vi "IMAQ OCR.vi"(0 "Image In":T1, 7 "error in":errorcluster) -> (21 "String (OCR/OCV 2)":string, 27 "error out":errorcluster)   [LabVIEW 2019]
doc: "This Vi contains the optical character recognition (OCR) which is the conversion of images containing text into machine-encoded text. In our case it is an image of licence plate, and OCR algorithm is reading it`s numbers."
uses:
  <vilib>/vision/Image Controls.llb/IMAQ Image.ctl
  <vilib>/vision/NI_Vision_Development_Module.lvlib
panel:
  # "Image In"
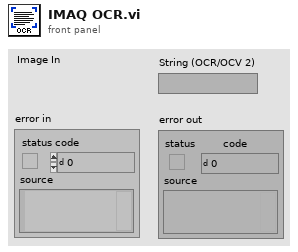
[diagram p1: front panel]
types:
  T1 = typedef "IMAQ Image.ctl" = refnum<image>
  T2 = cluster{"Threshold Data":cluster{"Method":enum16{"Fixed Range", "Uniform", "Linear", "Non Linear", "Local", "Color"}, "Looking for":u32, "Color Mode":u32, "Kernel Size":cluster{"Width":i32, "Height":i32}, "Ranges":cluster{"Min":i32, "Max":i32}[]}, "Reject Border":bool, "Number Of Erosions":i32, "Size & Spacing":cluster{"Segment Algorithm":u16, "Min Bounding Rect Width":i32, "Max Bounding Rect Width":i32, "Min Bounding Rect Height":i32, "Max Bounding Rect Height":i32, "Min Character Size":i32, "Max Character Size":i32, "Min Char Spacing":i32, "Max Horiz Element Spacing":i32, "Max Vert Element Spacing":i32, "Max Space Distance":i32}, "Read Options":cluster{"Read Strategy":i32, "Read Resolution":i32, "Scale Dependant":bool, "Aspect Ratio":i32, "Acceptance Level":i32, "Substitution Character":string, "MultiLine":bool}, "Valid Characters":cluster{"Pre-defined characters":i32, "User-defined characters":string}[], "Use Text Pattern":bool, "Orientation":u32, "# Lines Expected":u32, "Number of Blocks":i32}
  T3 = cluster{"Global Rectangle":i32[], "Contours":cluster{"ID":enum32{"External", "Internal"}, "Type":u32, "Coordinates":i32[]}[]}
  T4 = typedef "IMAQ OCR Session.ctl" = refnum<k1>
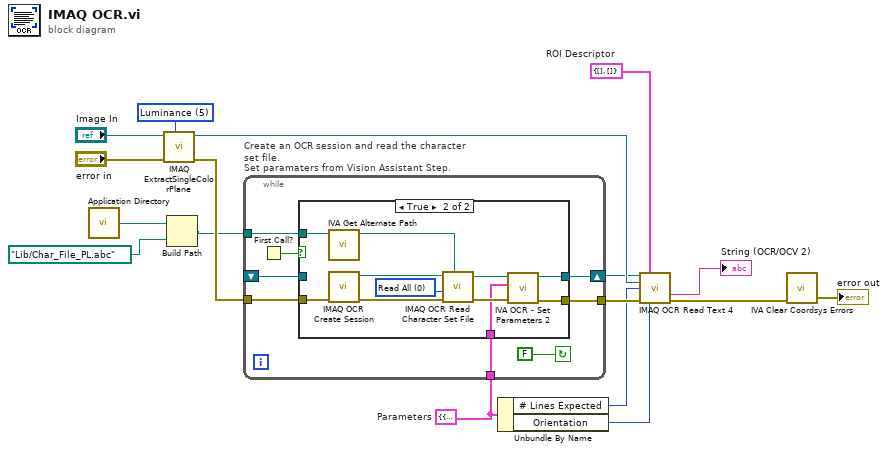
[diagram p0: block diagram]
diagram:
  w10 = T2 {"Threshold Data"={"Method"=enum."Uniform", "Looking for"=1, "Color Mode"=0, "Kernel Size"={"Width"=32, "Height"=32}, "Ranges"=[{"Min"=1, "Max"=255}]}, "Reject Border"=TRUE, "Number Of Erosions"=0, "Size & Spacing"={"Segment Algorithm"=0, "Min Bounding Rect Width"=1, "Max Bounding Rect Width"=65536, "Min Bounding Rect Height"=1, "Max Bounding Rect Height"=65536, "Min Character Size"=20, "Max Character Size"=65536, "Min Char Spacing"=1, "Max Horiz Element Spacing"=1, "Max Vert Element Spacing"=0, "Max Space Distance"=65536}, "Read Options"={"Read Strategy"=1, "Read Resolution"=2, "Scale Dependant"=FALSE, "Aspect Ratio"=400, "Acceptance Level"=700, "Substitution Character"="?", "MultiLine"=TRUE}, "Valid Characters"=[], "Use Text Pattern"=FALSE, "Orientation"=0, "# Lines Expected"=0, "Number of Blocks"=4}  # Parameters
  w12 = T3 {"Global Rectangle"=[], "Contours"=[]}  # ROI Descriptor
  w17 = 5 items=["Red", "Green", "Blue", "Hue", "Saturation", "Luminance", "Value", "Intensity"] ("Color Plane")
  n1 = call <vilib>:"Application Directory.vi"() -> ("Application Directory"=w3:path)
  n2 = call "IMAQ ExtractSingleColorPlane"("Color Plane"=w17, "error in (no error)"="error in", "Image Src"="Image In") -> ("error out"=w14:errorcluster, "Image Dst Out"=w11:T1)  [unwired: 1 in, 6 out]
  n3 = Build Path(base path=w3, name or relative path=path "Lib/Char_File_PL.abc") -> (appended path=w2:path)
  n4 = while "Create an OCR session and read the character set file.\nSet paramaters from Vision Assistant Step." {
    shift-right: [w22] -> w8
    shift-left: _ -> [w21]
    tunnel: w14 -> [w24]
    tunnel: w10 -> [w20]
    tunnel: w2 -> [w19]
    tunnel: [w18] -> w9
    stop <- FALSE continue-if-true
    n5 = First Call?() -> (First Call?: T/F=w23:bool)
    n6 = case shown="True" w23 {
      tunnel: w19 -> [_ w31]
      tunnel: w24 -> [w26 w35]
      tunnel: [w27 w33] -> w22
      tunnel: [w26 w32] -> w18
      tunnel: w20 -> [_ w28]
      tunnel: w21 -> [w27 _]
      frame False {
      }
      frame True {
        w36 = 0 items=["Read All", "Read Character Set Only", "Read Properties Only"] ("Read Options")
        n7 = call <vilib>:"IVA Get Alternate Path.vi"("Path In"=w31) -> ("Path Out"=w30:path)  [unwired: 10 out]
        n8 = call "IMAQ OCR Create Session"("error in (no error)"=w35) -> ("error out"=w37:errorcluster, "IMAQ OCR Session"=w38:T4)  [unwired: 9 out]
        n9 = call "IMAQ OCR Read Character Set File"("File Path"=w30, "error in (no error)"=w37, "Read Options"=w36, "IMAQ OCR Session"=w38) -> ("error out"=w34:errorcluster, "IMAQ OCR Session (dup)"=w29:T4)  [unwired: 1 in, 5 out]
        n10 = call <vilib>:"IVA OCR - Set Parameters 2.vi"("error in (no error)"=w34, "Parameters"=w28, "IMAQ OCR Session"=w29) -> ("error out"=w32:errorcluster, "IMAQ OCR Session Out"=w33:T4)  [unwired: 7 in]
      }
    }
  }
  n11 = Unbundle By Name(w10) -> ("# Lines Expected"=w6:u32, "Orientation"=w7:u32)
  n12 = call "IMAQ OCR Read Text 4"("IMAQ OCR Session"=w8, "ROI Descriptor"=w12, "Image"=w11, "Number of Lines Requested"=w6, "error in (no error)"=w9, "Orientation"=w7) -> ("Read String"=→"String (OCR/OCV 2)":string, "error out"=w5:errorcluster)  [unwired: 8 out]
  n13 = call <vilib>:"IVA Clear Coordsys Errors.vi"("error in (no error)"=w5) -> ("error out"=→"error out":errorcluster)  [unwired: 10 in]
